vi "Convert Kinect Data to r,theta.vi"(8 "error in (no error)":errorcluster, 9 "RD Data":cluster{"Depth":i32, "X":i32}, 10 "GN Data":cluster{"Depth":i32, "X":i32}, 11 "BL Data":cluster{"Depth":i32, "X":i32}) -> (0 "error out":errorcluster, 1 "Red":cluster{"R":dbl, "Theta":dbl}, 2 "Green":cluster{"R":dbl, "Theta":dbl}, 3 "Blue":cluster{"R":dbl, "Theta":dbl})   [LabVIEW 2009]
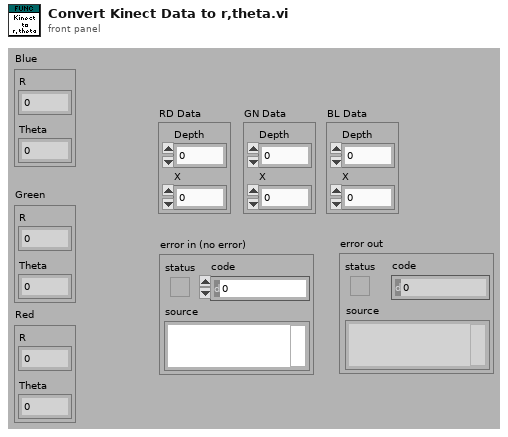
[diagram p1: front panel]
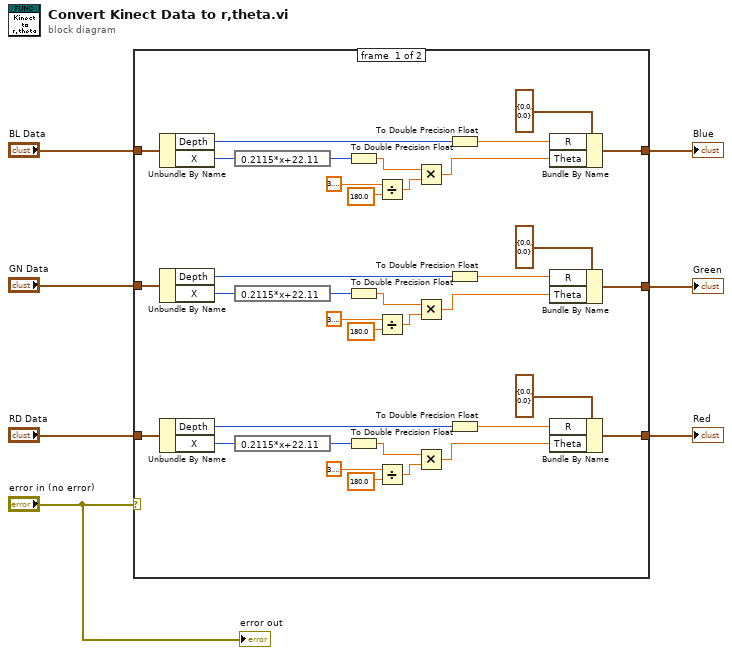
[diagram p0: block diagram]
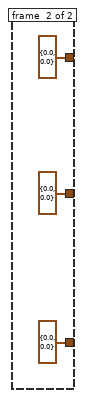
[diagram p2: hidden frame]
diagram:
  n1 = case shown="No Error" "error in (no error)" {
    tunnel: "BL Data" -> [w43 _]
    tunnel: [w40 cluster{"R":dbl, "Theta":dbl} {"R"=0.0, "Theta"=0.0} ("Blue")] -> w6
    tunnel: [w39 cluster{"R":dbl, "Theta":dbl} {"R"=0.0, "Theta"=0.0} ("Blue")] -> w5
    tunnel: [w36 cluster{"R":dbl, "Theta":dbl} {"R"=0.0, "Theta"=0.0} ("Blue")] -> w4
    tunnel: "GN Data" -> [w20 _]
    tunnel: "RD Data" -> [w10 _]
    frame #0 {
      n2 = Unbundle By Name(w43) -> ("Depth"=w41:i32, "X"=w35:i32)
      n3 = Unbundle By Name(w20) -> ("Depth"=w21:i32, "X"=w22:i32)
      n4 = Unbundle By Name(w10) -> ("Depth"=w17:i32, "X"=w16:i32)
      n5 = expression code="0.2115*x+22.11"(w35) -> (w30:i32)
      n6 = expression code="0.2115*x+22.11"(w22) -> (w26:i32)
      n7 = expression code="0.2115*x+22.11"(w16) -> (w12:i32)
      n8 = To Double Precision Float(number=w30) -> (double precision float=w29:dbl)
      n9 = To Double Precision Float(number=w26) -> (double precision float=w27:dbl)
      n10 = To Double Precision Float(number=w12) -> (double precision float=w11:dbl)
      n11 = Divide(x=3.141592653589793, y=180.0) -> (x/y=w31:dbl)
      n12 = Divide(x=3.141592653589793, y=180.0) -> (x/y=w25:dbl)
      n13 = Divide(x=3.141592653589793, y=180.0) -> (x/y=w13:dbl)
      n14 = Multiply(x=w29, y=w31) -> (x*y=w28:dbl)
      n15 = Multiply(x=w27, y=w25) -> (x*y=w18:dbl)
      n16 = Multiply(x=w11, y=w13) -> (x*y=w8:dbl)
      n17 = To Double Precision Float(number=w41) -> (double precision float=w34:dbl)
      n18 = To Double Precision Float(number=w21) -> (double precision float=w19:dbl)
      n19 = To Double Precision Float(number=w17) -> (double precision float=w9:dbl)
      n20 = Bundle By Name(cluster=cluster{"R":dbl, "Theta":dbl} {"R"=0.0, "Theta"=0.0} ("Blue"), "R"=w34, "Theta"=w28) -> (w40:cluster{"R":dbl, "Theta":dbl})
      n21 = Bundle By Name(cluster=cluster{"R":dbl, "Theta":dbl} {"R"=0.0, "Theta"=0.0} ("Blue"), "R"=w19, "Theta"=w18) -> (w39:cluster{"R":dbl, "Theta":dbl})
      n22 = Bundle By Name(cluster=cluster{"R":dbl, "Theta":dbl} {"R"=0.0, "Theta"=0.0} ("Blue"), "R"=w9, "Theta"=w8) -> (w36:cluster{"R":dbl, "Theta":dbl})
    }
    frame #1 {
    }
  }
  "Blue" <- w6
  "Green" <- w5
  "Red" <- w4
  "error out" <- "error in (no error)"
